vi "MakeAllMFCArrayCombos.vi"(11 "EvaluatedMFCs":T1[](array[typedef])) -> (2 "EveryCombination":T1[][](array[typedef]))   [LabVIEW 2016]
uses:
  MFCdescription.ctl
  MFCcapability.ctl
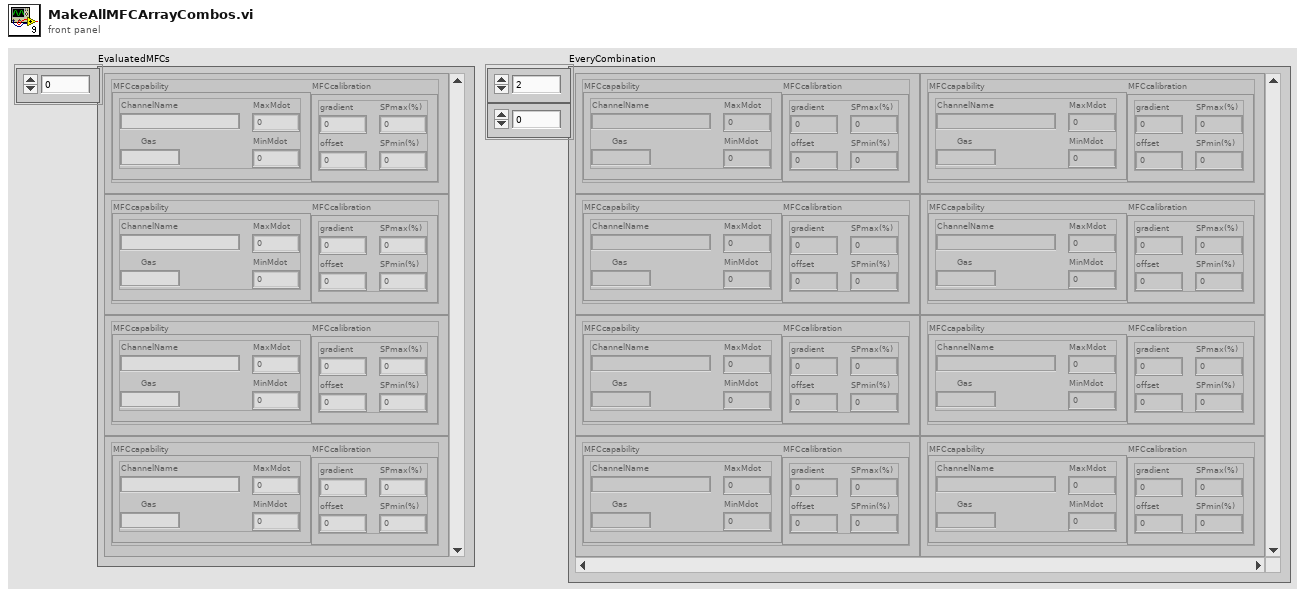
[diagram p1: front panel]
types:
  T1 = typedef "MFCdescription.ctl" = cluster{"MFCcapability":T2, "MFCcalibration":cluster{"gradient":dbl, "offset":dbl, "SPmin(%)":dbl, "SPmax(%)":dbl}}
  T2 = typedef "MFCcapability.ctl" = cluster{"ChannelName":string, "MinMdot":dbl, "MaxMdot":dbl, "Gas":string}
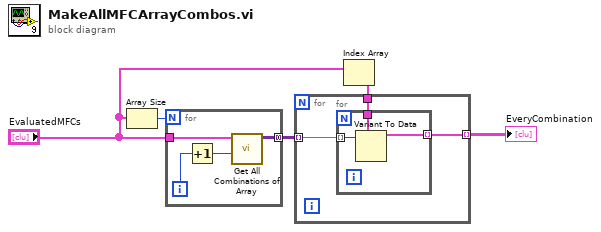
[diagram p0: block diagram]
diagram:
  n1 = Array Size(array="EvaluatedMFCs") -> (size(s)=w2:i32)
  n2 = for {
    N: w2 -> [_]
    tunnel: [w7] -> w3 mode=concatenating
    tunnel: "EvaluatedMFCs" -> [w6]
    i -> [w9]
    n3 = Increment(x=w9) -> (x+1=w8:i32)
    n4 = call "Get All Combinations of Array.vi"("Combination Length"=w8, "Array"=w6) -> ("Results Out"=w7:variant[][])  [unwired: 7 in, 2 out]
  }
  n5 = Index Array(array="EvaluatedMFCs") -> (element=w5:T1)  [unwired: 1 in]
  n6 = for {
    tunnel: w3 -> [w12] mode=indexing
    tunnel: [w11] -> w1 mode=indexing
    tunnel: w5 -> [w10]
    n7 = for {
      tunnel: w12 -> [w15] mode=indexing
      tunnel: [w13] -> w11 mode=indexing
      tunnel: w10 -> [w14]
      n8 = Variant To Data(type=w14, Variant=w15) -> (data=w13:T1)  [unwired: 1 in, 1 out]
    }
  }
  "EveryCombination" <- w1
